vi "try_Delimited String VIs.vi"() -> ()   [LabVIEW 2025]
panel:
  in  "String Array 2":string[](array[string])=["a", "b", "c", "d", "e", "f", "g"]
  out "Delimited String 2":string
  in  "Delimiter 2":string="-"
  out "String Array 1":string[](array[string])
  in  "Delimiter 1":string=","
  in  "Delimited String 1":string="A,B,C,D,E,F,G"
  # "Scenario\nThe 1D String Array to Delimited String.vi and Delimited String to 1D String Array.vi provide quick conversion between a string array and a delimited string\n\nInstructions\n1. To convert a Delimited String to a 1D String Array set the Delimiter 1 and Delimited String 1 controls, Run the VI and see the results in the String Array 1 Indicator \n2. To convert a 1D String Array to a Delimited String set the Delimiter 2 and String Array 2 controls, Run the VI and see the results in the Delimited String 2 Indicator \n\n2. Run the VI"
  # "1D String Array to Delimited String.vi"
  # "Delimited String to 1D String Array.vi"
  # "Close this VI when you are done with the demo."
  # "You do not need to save changes to this VI."
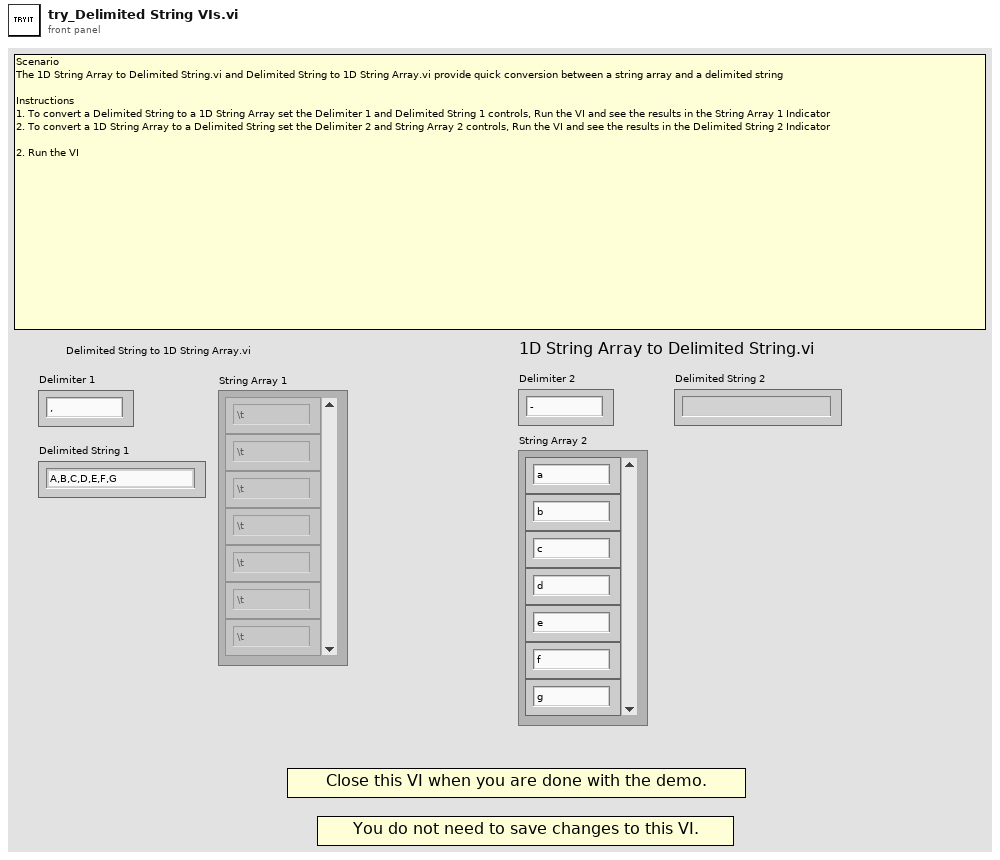
[diagram p1: front panel]
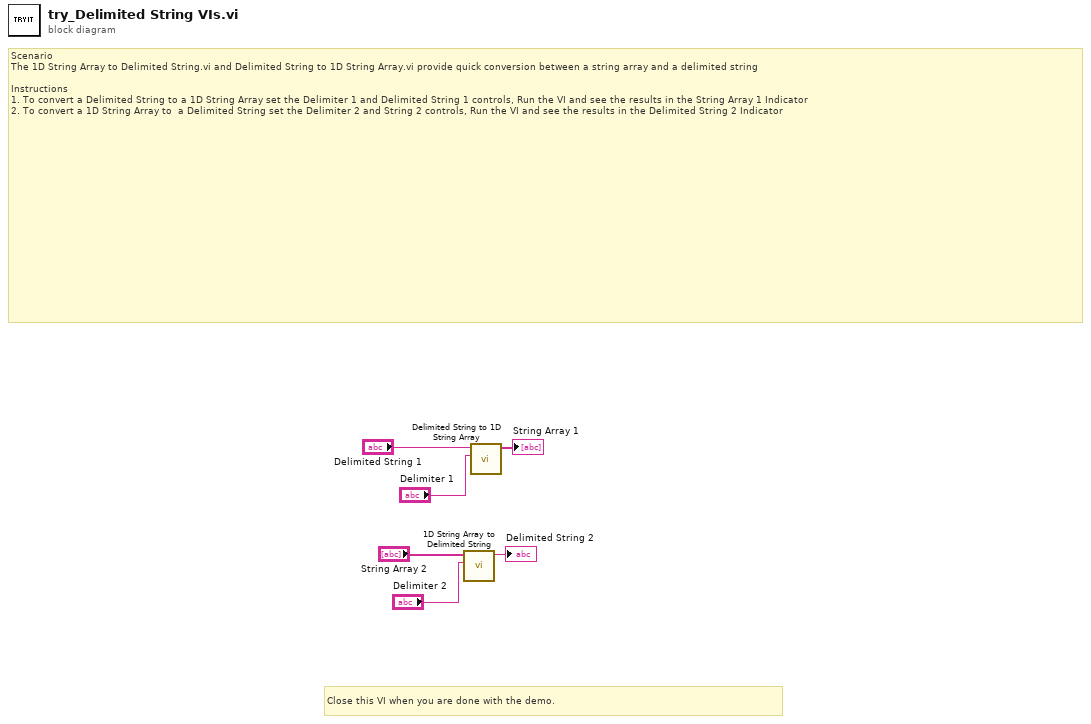
[diagram p0: block diagram]
diagram:
  # "Close this VI when you are done with the demo."
  # "Scenario\nThe 1D String Array to Delimited String.vi and Delimited String to 1D String Array.vi provide quick conversion between a string array and a delimited string \n\nInstructions\n1. To convert a Delimited String to a 1D String Array set the Delimiter 1 and Delimited String 1 controls, Run the VI and see the results in the String Array 1 Indicator \n2. To convert a 1D String Array to  a Delimited String set the Delimiter 2 and String 2 controls, Run the VI and see the results in the Delimited String 2 Indicator"
  n1 = call <vilib>:"1D String Array to Delimited String.vi"("delimiter"="Delimiter 2", "string array"="String Array 2") -> ("delimited string"=→"Delimited String 2":string)  [unwired: 9 in]
  n2 = call <vilib>:"Delimited String to 1D String Array.vi"("delimiter"="Delimiter 1", "delimited string"="Delimited String 1") -> ("string array"=→"String Array 1":string[])  [unwired: 9 in]
